vi "Open Drive Motors.vi"(8 "error in (no error)":errorcluster) -> (0 "error out":errorcluster)   [LabVIEW 2014]
uses:
  <vilib>/Rock Robotics/SystemInterfaces/DIO/FPGA_DIOPWMChannel.ctl
  <vilib>/Rock Robotics/WPI/SafetyOutput/WPI_SafetyOutputConfigMenu.ctl
  <vilib>/Rock Robotics/WPI/MotorControl/WPI_MotorControlOpen Talon.vi
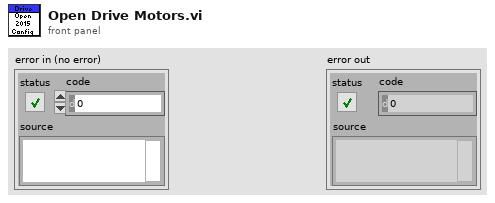
[diagram p1: front panel]
types:
  T1 = typedef "WPI_SafetyOutputConfigMenu.ctl" = enum16{"Enable", "Disable"}
  T2 = typedef "FPGA_DIOPWMChannel.ctl" = enum8{"PWM 0", "PWM 1", "PWM 2", "PWM 3", "PWM 4", "PWM 5", "PWM 6", "PWM 7", "PWM 8", "PWM 9", "PWM MXP 0", "PWM MXP 1", "PWM MXP 2", "PWM MXP 3", "PWM MXP 4", "PWM MXP 5", "PWM MXP 6", "PWM MXP 7", "PWM MXP 8", "PWM MXP 9", "Invalid"}
  T3 = typedef "WPI_MotorControlDeviceRef.ctl" = cluster{"DeviceStatus":errorcluster, "Type":T4, "PWM":cluster{"Controller":T5, "PWM Channel":T2, "DeadBand":T6}, "CAN":cluster{"Device Number":u8, "Control Mode":T7, "Semaphore":T8, "Max Vout":dbl, "TalonSRX Control Mode":T9}, "Invert":bool, "TransformRef":T10, "InvTransformRef":T10}
  T4 = typedef "WPI_MotorControlType.ctl" = enum16{"PWM", "CAN", "CANTalonSRX"}
  T5 = typedef "FPGA_TypedefDigitalModule.ctl" = enum16{"Controller 1"}
  T6 = typedef "WPI_PWMDeadband.ctl" = cluster{"Name":string, "maxPositivePwm":i32, "minPositivePwm":i32, "centerPwm":i32, "maxNegativePwm":i32, "minNegativePwm":i32, "angularRange":u16}
  T7 = typedef "WPI_CANJaguar_ControlMode.ctl" = enum8{"Percent VBus", "Current", "Speed", "Position", "Voltage"}
  T8 = typedef "Semaphore RefNum" = refnum<k1>
  T9 = typedef "WPI_CANTalonSRX_APIControlMode.ctl" = enum8{"Percent VBus", "Speed", "Position", "Slave", "Unchanged / Invalid"}
  T10 = typedef "WPI_PWMTransform_ConPane.ctl" = refnum<vi>
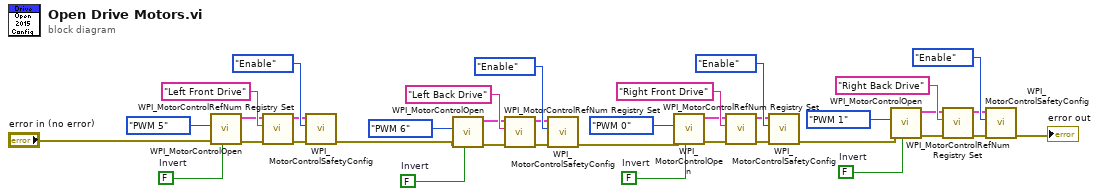
[diagram p0: block diagram]
diagram:
  w19 = FALSE  # Invert
  w20 = FALSE  # Invert
  w21 = FALSE  # Invert
  w18 = FALSE  # Invert
  n1 = call-poly <vilib>:"WPI_MotorControlOpen.vi"("Invert"=w19, "error in (no error)"="error in (no error)", "PWM Channel"=FPGA_DIOPWMChannel."PWM 5") -> ("error out"=w16:errorcluster, "MotorControlDeviceRef"=w17:T3)  [unwired: 7 in]
  n2 = call <vilib>:"WPI_MotorControlRefNum Registry Set.vi"("error in (no error)"=w16, "refnum name"="Left Front Drive", "MotorControlDevRef"=w17) -> ("error out"=w30:errorcluster, "MotorControlDevRef"=w31:T3)  [unwired: 7 in]
  n3 = call <vilib>:"WPI_MotorControlSafetyConfig.vi"("error in (no error)"=w30, "mode"=WPI_SafetyOutputConfigMenu."Enable", "MotorControlDevRef"=w31) -> ("error out"=w4:errorcluster)  [unwired: 7 in, 1 out]
  n4 = call-poly <vilib>:"WPI_MotorControlOpen.vi"("Invert"=w20, "error in (no error)"=w4, "PWM Channel"=FPGA_DIOPWMChannel."PWM 6") -> ("error out"=w14:errorcluster, "MotorControlDeviceRef"=w15:T3)  [unwired: 7 in]
  n5 = call <vilib>:"WPI_MotorControlRefNum Registry Set.vi"("error in (no error)"=w14, "refnum name"="Left Back Drive", "MotorControlDevRef"=w15) -> ("error out"=w32:errorcluster, "MotorControlDevRef"=w33:T3)  [unwired: 7 in]
  n6 = call <vilib>:"WPI_MotorControlSafetyConfig.vi"("error in (no error)"=w32, "mode"=WPI_SafetyOutputConfigMenu."Enable", "MotorControlDevRef"=w33) -> ("error out"=w3:errorcluster)  [unwired: 7 in, 1 out]
  n7 = call-poly <vilib>:"WPI_MotorControlOpen.vi"("Invert"=w21, "error in (no error)"=w3, "PWM Channel"=FPGA_DIOPWMChannel."PWM 0") -> ("error out"=w12:errorcluster, "MotorControlDeviceRef"=w13:T3)  [unwired: 7 in]
  n8 = call <vilib>:"WPI_MotorControlRefNum Registry Set.vi"("error in (no error)"=w12, "refnum name"="Right Front Drive", "MotorControlDevRef"=w13) -> ("error out"=w28:errorcluster, "MotorControlDevRef"=w29:T3)  [unwired: 7 in]
  n9 = call <vilib>:"WPI_MotorControlSafetyConfig.vi"("error in (no error)"=w28, "mode"=WPI_SafetyOutputConfigMenu."Enable", "MotorControlDevRef"=w29) -> ("error out"=w2:errorcluster)  [unwired: 7 in, 1 out]
  n10 = call-poly <vilib>:"WPI_MotorControlOpen.vi"("Invert"=w18, "error in (no error)"=w2, "PWM Channel"=FPGA_DIOPWMChannel."PWM 1") -> ("error out"=w10:errorcluster, "MotorControlDeviceRef"=w11:T3)  [unwired: 7 in]
  n11 = call <vilib>:"WPI_MotorControlRefNum Registry Set.vi"("error in (no error)"=w10, "refnum name"="Right Back Drive", "MotorControlDevRef"=w11) -> ("error out"=w26:errorcluster, "MotorControlDevRef"=w27:T3)  [unwired: 7 in]
  n12 = call <vilib>:"WPI_MotorControlSafetyConfig.vi"("error in (no error)"=w26, "mode"=WPI_SafetyOutputConfigMenu."Enable", "MotorControlDevRef"=w27) -> ("error out"=→"error out":errorcluster)  [unwired: 7 in, 1 out]
